vi "查找文件序号最大值.vi"(11 "存储路径":path=path "D:/") -> (3 "文件索引最大值+1":string)   [LabVIEW 2020]
panel:
  out "文件名":string[](array[string])
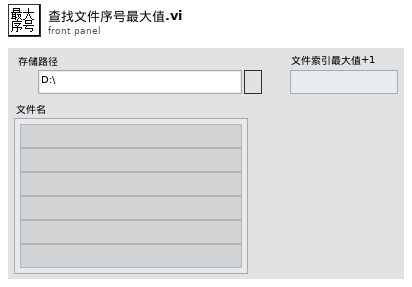
[diagram p1: front panel]
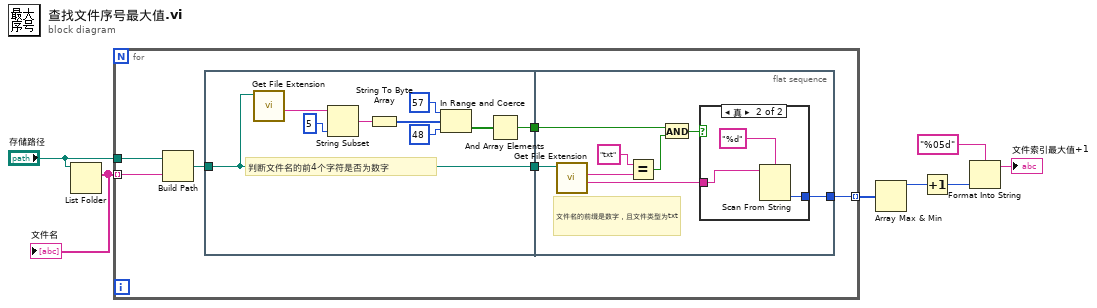
[diagram p0: block diagram]
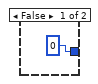
[diagram p2: hidden frame]
diagram:
  n1 = List Folder(path="存储路径") -> (filenames=w7:string[])  [unwired: 3 in, 3 out]
  "文件名" <- w7
  n2 = for {
    tunnel: w7 -> [w10] mode=indexing
    tunnel: [w11] -> w6 mode=indexing
    tunnel: "存储路径" -> [w8]
    n3 = Build Path(base path=w8, name or relative path=w10) -> (appended path=w9:path)
    n4 = flat-sequence {
      tunnel: w9 -> [w14]
      tunnel: [w14] -> w13
      tunnel: [w15] -> w12
      tunnel: w13 -> [w29]
      tunnel: w12 -> [w24]
      tunnel: [w30] -> w11
      frame #0 {
        # "判断文件名的前4个字符是否为数字"
        n5 = call <vilib>:"Get File Extension.vi"("file"=w14) -> ("filename without extension"=w16:string)  [unwired: 6 in, 4 out]
        n6 = String Subset(string=w16, length (rest)=5 ("长度（剩余）")) -> (substring=w21:string)  [unwired: 1 in]
        n7 = String To Byte Array(string=w21) -> (unsigned byte array=w18:u8[])
        n8 = In Range and Coerce(upper limit=u8 57, x=w18, lower limit=u8 48) -> (In Range?=w17:bool[])  [unwired: 1 out]
        n9 = And Array Elements(Boolean array=w17) -> (logical AND=w15:bool)
      }
      frame #1 {
        # "文件名的前缀是数字，且文件类型为txt"
        n10 = call <vilib>:"Get File Extension.vi"("file"=w29) -> ("filename without extension"=w28:string, "lowercase file extension"=w27:string)  [unwired: 6 in, 3 out]
        n11 = Equal?(x="txt", y=w27) -> (x = y?=w25:bool)
        n12 = And(x=w24, y=w25) -> (x .and. y?=w23:bool)
        n13 = case shown="真" w23 {
          tunnel: [0 w33] -> w30
          tunnel: w28 -> [_ w32]
          frame False {
          }
          frame True {
            n14 = Scan From String(format string="%d" ("格式字符串"), input string=w32) -> (output 1=w33:i32)  [unwired: 3 in, 3 out]
          }
        }
      }
    }
  }
  n15 = Array Max & Min(array=w6) -> (max value=w2:i32)  [unwired: 3 out]
  n16 = Increment(x=w2) -> (x+1=w3:i32)
  n17 = Format Into String(format string="%05d" ("格式字符串"), w3) -> (resulting string=→"文件索引最大值+1":string)  [unwired: 2 in, 1 out]
